vi "9403_UI.vi"(8 "error in (no error)":errorcluster, 11 "Node Ptr":T1 format="%.0x") -> (0 "error out":errorcluster)   [LabVIEW 2020, in "Modules.lvlib" / "9403.lvclass"]
uses:
  9403.lvclass
  <vilib>/NI VeriStand/Custom Device API/Custom Device Item Ref.ctl
  RSI Module/SubPanel Command.ctl
  C:/Users/nitest/Desktop/Git 2020/niveristand-scan-engine-module-libraries/Source/RSI Module/RSI Module.lvclass
  9403.lvclass/9403.ctl
  RSI Module/RSI Module.lvclass
  <vilib>/NI VeriStand/Custom Device API/Custom Device API.lvlib
panel:
  out "Line Directions":enum16{"Input", "Output"}[](array[ring])
  out "_Selected Channel(s) Settings Label":string="Selected Channel(s) Settings"
  in  "Channels":i32[](listbox)=[29]
  in  "LineDirectionVal":u32(ring)=1 caption="Initial Line Direction" items=["Input", "Output"]
  in  "BadLineDirectionVal":u32(ring) caption="Initial Line Direction" items=["Input", "Output", "X"]
  in  "SubPanel Event":refnum<user-event>
  in  "Header":cluster{"Section Name":string}={"Section Name"="NI 9403 Settings"}
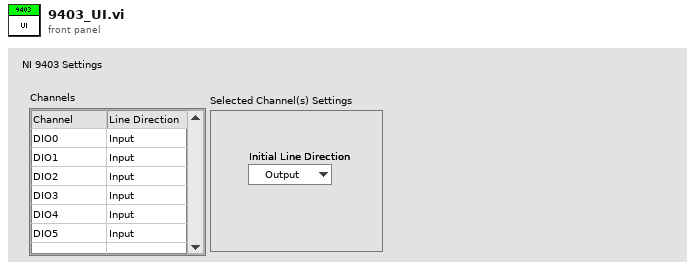
[diagram p1: front panel]
types:
  T1 = typedef "Custom Device API.lvlib/Custom Device Item Ref.ctl" = u64
  T2 = typedef "Modules.lvlib/RSI Module.lvclass/Module Models.ctl" = enum16{"Empty", "NI 9201", "NI 9203", "NI 9205", "NI 9206", "NI 9207", "NI 9208", "NI 9209", "NI 9210", "NI 9211", "NI 9212", "NI 9213", "NI 9214", "NI 9215", "NI 9216", "NI 9217", "NI 9219", "NI 9220", "NI 9221", "NI 9222", "NI 9223", "NI 9224", "NI 9225", "NI 9226", "NI 9227", "NI 9228", "NI 9229", "NI 9233", "NI 9234", "NI 9235", "NI 9236", "NI 9237", "NI 9239", "NI 9242", "NI 9244", "NI 9253", "NI 9263", "NI 9264", "NI 9265", "NI 9266", "NI 9269", "NI 9344", "NI 9350", "NI 9375", "NI 9401", "NI 9402", "NI 9403", "NI 9411", "NI 9421", "NI 9422", "NI 9423", "NI 9425", "NI 9426", "NI 9435", "NI 9436", "NI 9437", "NI 9472", "NI 9474", "NI 9475", "NI 9476", "NI 9477", "NI 9478", "NI 9481", "NI 9482", "NI 9485"}
  T3 = typedef "Custom Device API.lvlib/Custom Device Item Info.ctl" = cluster{"Name":string, "Is Channel":bool, "GUID":string, "Is Waveform":bool}
  T4 = typedef "Modules.lvlib/RSI Module.lvclass/SubPanel Command.ctl" = enum16{"Stop"}
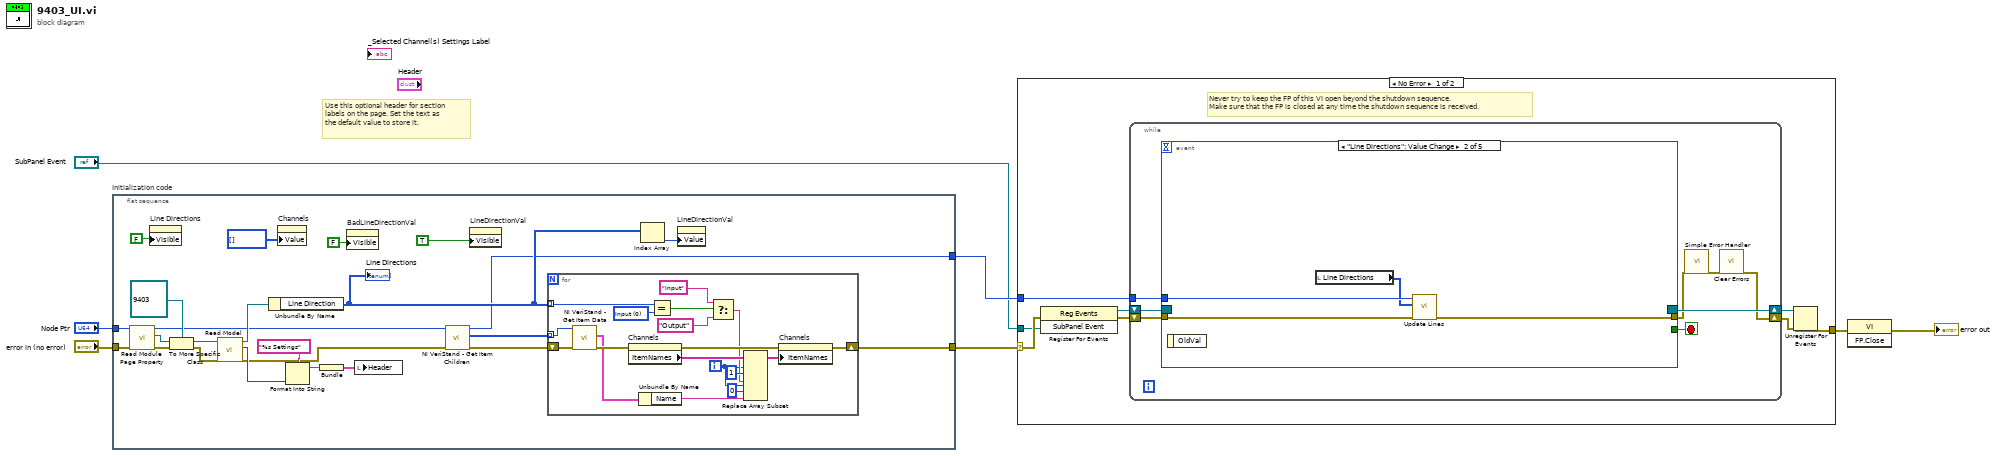
[diagram p0: block diagram]
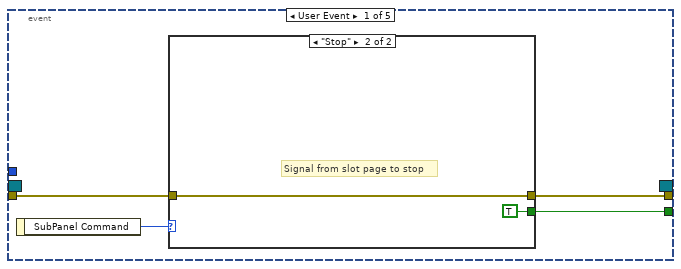
[diagram p2: hidden frame]
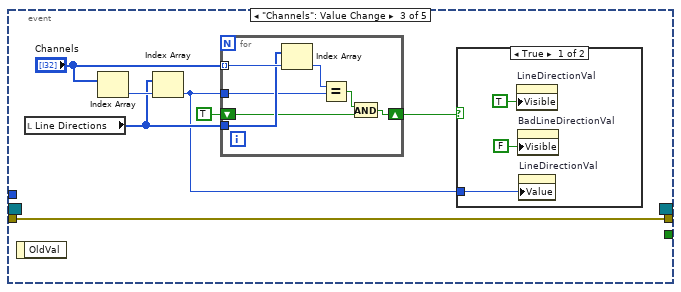
[diagram p4: hidden frame]
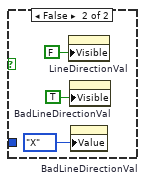
[diagram p5: hidden frame]
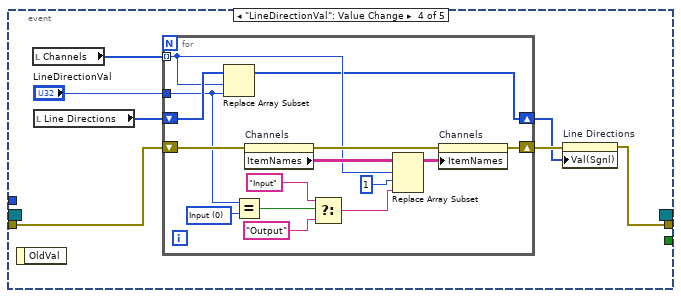
[diagram p6: hidden frame]
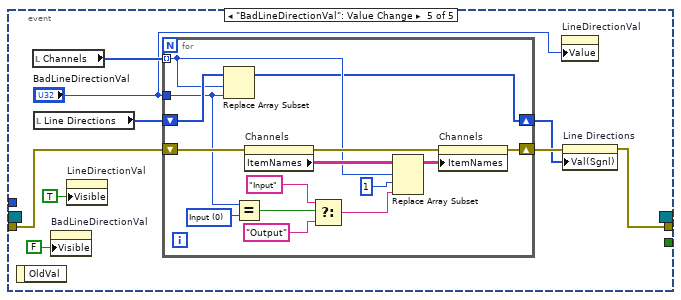
[diagram p7: hidden frame]
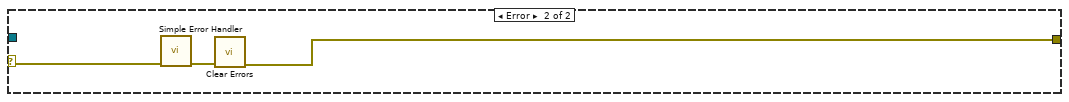
[diagram p8: hidden frame]
diagram:
  # "Use this optional header for section labels on the page. Set the text as the default value to store it."
  n1 = flat-sequence "Initialization code" {
    tunnel: "error in (no error)" -> [w30]
    tunnel: "Node Ptr" -> [w31]
    tunnel: [w14] -> w1
    tunnel: [w10] -> w4
    frame #0 {
      n2 = call "Read Module Page Property.vi"("error in (no error)"=w30, "Node Ptr In"=w31) -> ("error out"=w29:errorcluster, "RSI Module"=w27:refnum<class "RSI Module.lvclass">, "Node Ptr Out"=w11:T1)  [unwired: 7 in]
      n3 = property on="Line Directions" class="Arr (strict)"("Visible"=FALSE) -> ()  [unwired: 2 in, 2 out]
      n4 = To More Specific Class(target class=refnum<class "9403.lvclass"> refnum ("9205 in"), reference=w27, error in=w29) -> (specific class reference=w26:refnum<class "9403.lvclass">, error out=w25:errorcluster)
      n5 = call "Read Model.vi"("error in (no error)"=w25, "RSI Module in"=w26) -> ("error out"=w12:errorcluster, "Model"=w23:T2, "RSI Module out"=w20:refnum<class "9403.lvclass">)  [unwired: 7 in]
      n6 = Unbundle By Name(w20) -> ("Line Direction"=w13:u32[])
      "Line Directions" <- w13
      n7 = property on="Channels" class="MCListbox (strict)"("Value"=i32[] [] ("Channels")) -> ()  [unwired: 2 in, 2 out]
      n8 = Format Into String(format string="%s Settings", w23) -> (resulting string=w21:string)  [unwired: 2 in, 1 out]
      n9 = Bundle(w21) -> (w24:cluster{string})  [unwired: 1 in]
      n10 = property on="BadLineDirectionVal" class="Ring (strict)"("Visible"=FALSE) -> ()  [unwired: 2 in, 2 out]
      n11 = local write "Header"(w24) -> ()
      n12 = call <vilib>:"NI VeriStand - Get Item Children.vi"("error in (no error)"=w12, "Item Ref in"=w11) -> ("error out"=w9:errorcluster, "Child Refs"=w8:T1[], "Item Ref out"=w10:T1)  [unwired: 6 in, 1 out]
      n13 = property on="LineDirectionVal" class="Ring (strict)"("Visible"=TRUE) -> ()  [unwired: 2 in, 2 out]
      n14 = for {
        shift-right: [w41] -> w14
        shift-left: w9 -> [w38]
        tunnel: w13 -> [w47] mode=indexing
        tunnel: w8 -> [w36] mode=indexing
        i -> [w33]
        w46 = u32 0 items=["Input", "Output"] ("DIO9:Line direction")
        n15 = call <vilib>:"NI VeriStand - Get Item Data.vi"("error in (no error)"=w38, "Item Ref in"=w36) -> ("error out"=w37:errorcluster, "Item Info"=w35:T3)  [unwired: 6 in, 2 out]
        n16 = property on="Channels" class="MCListbox (strict)"(error in=w37) -> (error out=w42:errorcluster, "ItemNames"=w49:string[][])  [unwired: 1 in, 1 out]
        n17 = Unbundle By Name(w35) -> ("Name"=w32:string)
        n18 = Equal?(x=w47, y=w46) -> (x = y?=w45:bool)
        n19 = Select(t="Input", s=w45, f="Output") -> (s? t:f=w39:string)
        n20 = Replace Array Subset(array=w49, new element #1=w39, index (row) #1=w33, index (col) #1=1 ("disabled index (col)"), new element #2=w32, index (row) #2=w33, index (col) #2=0 ("disabled index (col)")) -> (w40:string[][])
        n21 = property on="Channels" class="MCListbox (strict)"(error in=w42, "ItemNames"=w40) -> (error out=w41:errorcluster)  [unwired: 1 in, 1 out]
      }
      n22 = Index Array(array=w13) -> (element=w15:u32)  [unwired: 1 in]
      n23 = property on="LineDirectionVal" class="Ring (strict)"("Value"=w15) -> ()  [unwired: 2 in, 2 out]
    }
  }
  n24 = case shown="No Error" w1 {
    selector: w1 -> [w51 w145]
    tunnel: [w55 w143] -> w7
    tunnel: w4 -> [w52 _]
    tunnel: "SubPanel Event" -> [w50 _]
    frame No Error {
      # "Never try to keep the FP of this VI open beyond the shutdown sequence.\nMake sure that the FP is closed at any time the shutdown sequence is received."
      n25 = register-events(error in=w51, w50) -> (reference out=w53:refnum<event-registration>, error out=w54:errorcluster)  [unwired: 1 in]
      n26 = while {
        tunnel: w52 -> [w61]
        shift-right: [w58] -> w56
        shift-left: w54 -> [w64]
        shift-right: [w65] -> w57
        shift-left: w53 -> [w63]
        stop <- w62 stop-if-true
        n27 = event shown="[1] \"Line Directions\": Value Change" {
          selector: w63 -> [_ _ _ _ _]
          dyn-events: [_ _ _ _ _] -> w65
          timeout: _ -> [_ _ _ _ _]
          tunnel: w64 -> [w68 w76 w77 w100 w125]
          tunnel: [w67 _ _ _ _] -> w62
          tunnel: [w66 w75 w77 w97 w122] -> w60
          tunnel: w61 -> [_ w74 _ _ _]
          event User Event {
            n28 = event-data() -> ("SubPanel Command"=w69:T4)  [unwired: 1 out]
            n29 = case shown="\"Stop\"" w69 {
              tunnel: w68 -> [w70 w71]
              tunnel: [w70 w71] -> w66
              tunnel: [_ TRUE] -> w67
              frame Default {
              }
              frame "Stop" {
                # "Signal from slot page to stop"
              }
            }
          }
          event "Line Directions": Value Change {
            n30 = event-data() -> ()  [unwired: 2 out]
            n31 = local read "Line Directions"() -> (w73:enum16{"Input", "Output"}[])
            n32 = call "Update Lines.vi"("error in (no error)"=w76, "Line Directions"=w73, "Node Ptr in"=w74) -> ("error out"=w75:errorcluster)  [unwired: 7 in, 1 out]
          }
          event "Channels": Value Change {
            n33 = event-data() -> ()  [unwired: 2 out]
            n34 = local read "Line Directions"() -> (w80:enum16{"Input", "Output"}[])
            n35 = Index Array(array="Channels") -> (element=w83:i32)  [unwired: 1 in]
            n36 = Index Array(array=w80, index=w83) -> (element=w78:enum16{"Input", "Output"})
            n37 = for {
              tunnel: "Channels" -> [w87] mode=indexing
              shift-right: [w88] -> w79
              shift-left: TRUE -> [w84]
              tunnel: w78 -> [w85]
              tunnel: w80 -> [w86]
              n38 = Index Array(array=w86, index=w87) -> (element=w89:enum16{"Input", "Output"})
              n39 = Equal?(x=w89, y=w85) -> (x = y?=w90:bool)
              n40 = And(x=w90, y=w84) -> (x .and. y?=w88:bool)
            }
            n41 = case shown="True" w79 {
              tunnel: w78 -> [w91 _]
              frame True {
                n42 = property on="LineDirectionVal" class="Ring (strict)"("Visible"=TRUE) -> ()  [unwired: 2 in, 2 out]
                n43 = property on="BadLineDirectionVal" class="Ring (strict)"("Visible"=FALSE) -> ()  [unwired: 2 in, 2 out]
                n44 = property on="LineDirectionVal" class="Ring (strict)"("Value"=w91) -> ()  [unwired: 2 in, 2 out]
              }
              frame False {
                n45 = property on="LineDirectionVal" class="Ring (strict)"("Visible"=FALSE) -> ()  [unwired: 2 in, 2 out]
                n46 = property on="BadLineDirectionVal" class="Ring (strict)"("Visible"=TRUE) -> ()  [unwired: 2 in, 2 out]
                n47 = property on="BadLineDirectionVal" class="Ring (strict)"("Value"=enum16{"0", "1", "X"}."X" ("BadNumOutputSyncRegs")) -> ()  [unwired: 2 in, 2 out]
              }
            }
          }
          event "LineDirectionVal": Value Change {
            n48 = event-data() -> ()  [unwired: 2 out]
            n49 = local read "Channels"() -> (w103:i32[])
            n50 = local read "Line Directions"() -> (w101:enum16{"Input", "Output"}[])
            n51 = for {
              tunnel: w103 -> [w106] mode=indexing
              tunnel: "LineDirectionVal" -> [w105]
              shift-right: [w104] -> w98
              shift-left: w101 -> [w118]
              shift-right: [w107] -> w99
              shift-left: w100 -> [w108]
              w111 = u32 0 items=["Input", "Output"] ("DIO9:Line direction")
              n52 = Replace Array Subset(array=w118, new element=w105, index=w106) -> (w104:enum16{"Input", "Output"}[])
              n53 = Equal?(x=w105, y=w111) -> (x = y?=w112:bool)
              n54 = property on="Channels" class="MCListbox (strict)"(error in=w108) -> (error out=w115:errorcluster, "ItemNames"=w109:string[][])  [unwired: 1 in, 1 out]
              n55 = Select(t="Input", s=w112, f="Output") -> (s? t:f=w117:string)
              n56 = Replace Array Subset(array=w109, new element=w117, index (row)=w106, index (col)=1 ("disabled index (col)")) -> (w116:string[][])
              n57 = property on="Channels" class="MCListbox (strict)"(error in=w115, "ItemNames"=w116) -> (error out=w107:errorcluster)  [unwired: 1 in, 1 out]
            }
            n58 = property on="Line Directions" class="Arr (strict)"(error in=w99, "Val(Sgnl)"=w98) -> (error out=w97:errorcluster)  [unwired: 1 in, 1 out]
          }
          event "BadLineDirectionVal": Value Change {
            n59 = event-data() -> ()  [unwired: 2 out]
            n60 = local read "Channels"() -> (w127:i32[])
            n61 = local read "Line Directions"() -> (w126:enum16{"Input", "Output"}[])
            n62 = property on="BadLineDirectionVal" class="Ring (strict)"("Visible"=FALSE) -> ()  [unwired: 2 in, 2 out]
            n63 = property on="LineDirectionVal" class="Ring (strict)"("Visible"=TRUE) -> ()  [unwired: 2 in, 2 out]
            n64 = for {
              tunnel: w127 -> [w130] mode=indexing
              tunnel: "BadLineDirectionVal" -> [w129]
              shift-right: [w128] -> w123
              shift-left: w126 -> [w142]
              shift-right: [w131] -> w124
              shift-left: w125 -> [w132]
              w135 = u32 0 items=["Input", "Output"] ("DIO9:Line direction")
              n65 = Replace Array Subset(array=w142, new element=w129, index=w130) -> (w128:enum16{"Input", "Output"}[])
              n66 = Equal?(x=w129, y=w135) -> (x = y?=w136:bool)
              n67 = property on="Channels" class="MCListbox (strict)"(error in=w132) -> (error out=w139:errorcluster, "ItemNames"=w133:string[][])  [unwired: 1 in, 1 out]
              n68 = Select(t="Input", s=w136, f="Output") -> (s? t:f=w141:string)
              n69 = Replace Array Subset(array=w133, new element=w141, index (row)=w130, index (col)=1 ("disabled index (col)")) -> (w140:string[][])
              n70 = property on="Channels" class="MCListbox (strict)"(error in=w139, "ItemNames"=w140) -> (error out=w131:errorcluster)  [unwired: 1 in, 1 out]
            }
            n71 = property on="LineDirectionVal" class="Ring (strict)"("Value"="BadLineDirectionVal") -> ()  [unwired: 2 in, 2 out]
            n72 = property on="Line Directions" class="Arr (strict)"(error in=w124, "Val(Sgnl)"=w123) -> (error out=w122:errorcluster)  [unwired: 1 in, 1 out]
          }
        }
        n73 = call <vilib>:"Simple Error Handler.vi"("error in (no error)"=w60) -> ("error out"=w59:errorcluster)  [unwired: 1 in, 7 out]
        n74 = call <vilib>:"Clear Errors.vi"("error in (no error)"=w59) -> ("error out"=w58:errorcluster)  [unwired: 1 in, 5 out]
      }
      n75 = Unregister For Events(event registration refnum=w57, error in=w56) -> (error out=w55:errorcluster)
    }
    frame Error {
      n76 = call <vilib>:"Simple Error Handler.vi"("error in (no error)"=w145) -> ("error out"=w144:errorcluster)  [unwired: 1 in, 7 out]
      n77 = call <vilib>:"Clear Errors.vi"("error in (no error)"=w144) -> ("error out"=w143:errorcluster)  [unwired: 1 in, 5 out]
    }
  }
  n78 = invoke class="VI" method="FP.Close"(error in=w7) -> (error out=→"error out":errorcluster)  [unwired: 2 in, 2 out]
